vi "DESTROY UE.vi"(8 "error in (no error)":errorcluster, 11 "DATABASE in":refnum<class "DATABASE.lvclass">) -> (0 "error out":errorcluster, 3 "DATABASE out":refnum<class "DATABASE.lvclass">)   [LabVIEW 2019, in "DATABASE.lvlib" / "DATABASE.lvclass"]
uses:
  DATABASE.lvclass
  DATABASE.lvclass/DATABASE.ctl
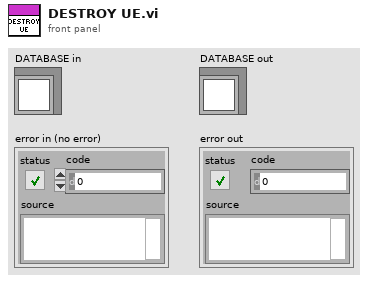
[diagram p1: front panel]
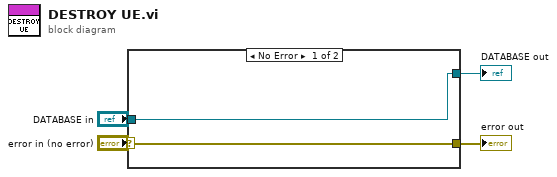
[diagram p0: block diagram]
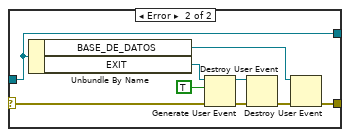
[diagram p2: hidden frame]
diagram:
  n1 = case shown="No Error" "error in (no error)" {
    selector: "error in (no error)" -> [w6 w12]
    tunnel: [w6 w7] -> w2
    tunnel: [w5 w8] -> w3
    tunnel: "DATABASE in" -> [w5 w8]
    frame No Error {
    }
    frame Error {
      n2 = Unbundle By Name(w8) -> ("BASE_DE_DATOS"=w9:refnum<user-event>, "EXIT"=w15:refnum<user-event>)
      n3 = Generate User Event(user event=w15, event data cluster=TRUE ("event data"), error in=w12) -> (user event out=w13:refnum<user-event>, error out=w11:errorcluster)  [unwired: 1 in]
      n4 = Destroy User Event(user event=w13, error in=w11) -> (error out=w10:errorcluster)
      n5 = Destroy User Event(user event=w9, error in=w10) -> (error out=w7:errorcluster)
    }
  }
  "DATABASE out" <- w3
  "error out" <- w2
